vi "Lithography.vi"(8 "Enum":enum16{"Stop", "Start"}(ring), 10 "error in (no error)":errorcluster) -> (2 "error out":errorcluster)   [LabVIEW 2014]
panel:
  in  "AutoItX3Lib.IAutoItX3":refnum<k7>
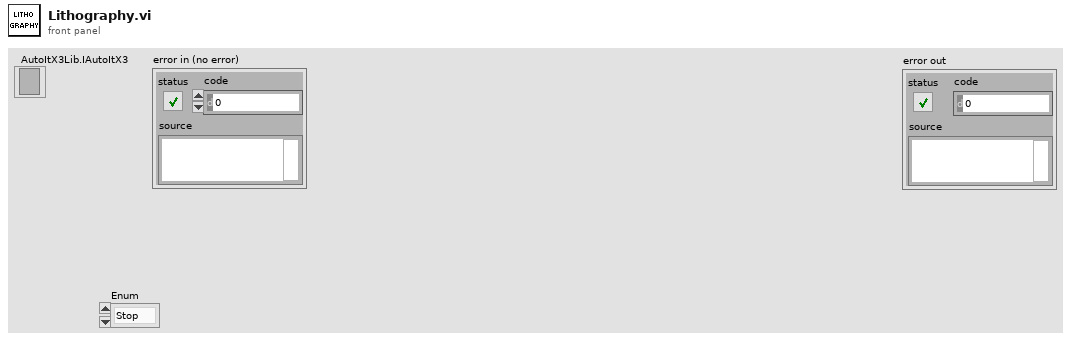
[diagram p1: front panel]
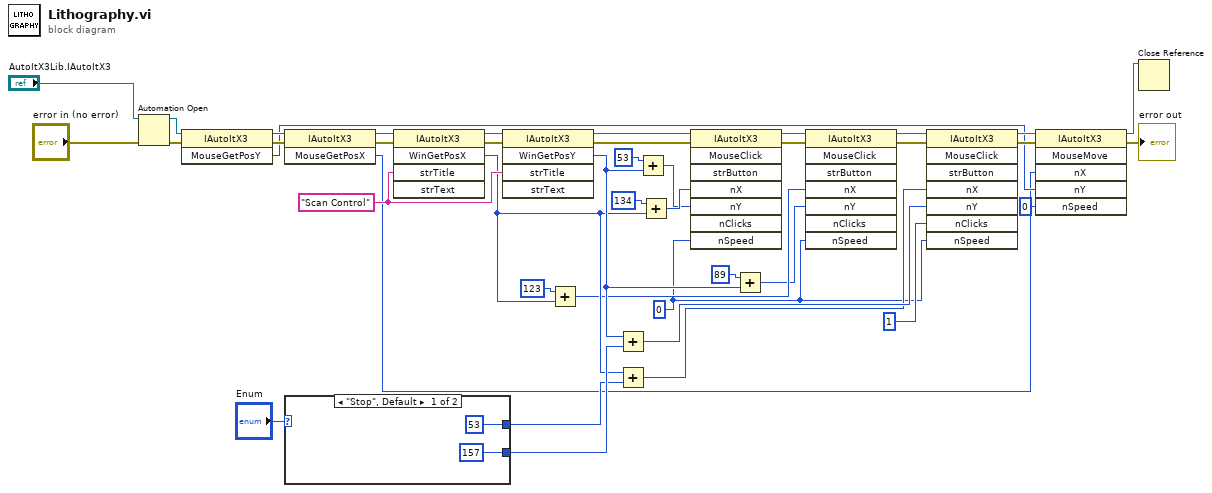
[diagram p0: block diagram]
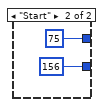
[diagram p2: hidden frame]
diagram:
  w10 = 0 ("nSpeed")
  w37 = "Scan Control" ("strTitle")
  n1 = Automation Open(error in (no error)="error in (no error)", Automation Refnum="AutoItX3Lib.IAutoItX3") -> (Automation Refnum=w39:refnum<k7>, error out=w4:errorcluster)  [unwired: 2 in]
  n2 = invoke class="IAutoItX3" method="MouseGetPosY"(reference=w39, error in=w4) -> (reference out=w8:refnum<k7>, error out=w5:errorcluster, "MouseGetPosY"=w3:i32)  [unwired: 1 in]
  n3 = invoke class="IAutoItX3" method="MouseGetPosX"(reference=w8, error in=w5) -> (reference out=w9:refnum<k7>, error out=w6:errorcluster, "MouseGetPosX"=w2:i32)  [unwired: 1 in]
  n4 = case shown="\"Stop\", Default" "Enum" {
    tunnel: [157 ("y") 156 ("y")] -> w33
    tunnel: [53 ("y") 75 ("y")] -> w29
    frame "Stop", Default {
    }
    frame "Start" {
    }
  }
  n5 = invoke class="IAutoItX3" method="WinGetPosX"(reference=w9, error in=w6, "strTitle"=w37) -> (reference out=w35:refnum<k7>, error out=w36:errorcluster, "WinGetPosX"=w19:i32)  [unwired: 2 in, 2 out]
  n6 = invoke class="IAutoItX3" method="WinGetPosY"(reference=w35, error in=w36, "strTitle"=w37) -> (reference out=w40:refnum<k7>, error out=w23:errorcluster, "WinGetPosY"=w20:i32)  [unwired: 2 in, 2 out]
  n7 = Add(x=123, y=w19) -> (x+y=w16:i32)
  n8 = Add(x=w20, y=w33) -> (x+y=w34:i32)
  n9 = Add(x=w19, y=w29) -> (x+y=w30:i32)
  n10 = Add(x=53, y=w20) -> (x+y=w17:i32)
  n11 = Add(x=134, y=w19) -> (x+y=w18:i32)
  n12 = invoke class="IAutoItX3" method="MouseClick"(reference=w40, error in=w23, "nX"=w18, "nY"=w17, "nSpeed"=w10) -> (reference out=w25:refnum<k7>, error out=w22:errorcluster)  [unwired: 3 in, 6 out]
  n13 = Add(x=89, y=w20) -> (x+y=w15:i32)
  n14 = invoke class="IAutoItX3" method="MouseClick"(reference=w25, error in=w22, "nX"=w16, "nY"=w15, "nSpeed"=w10) -> (reference out=w24:refnum<k7>, error out=w21:errorcluster)  [unwired: 3 in, 6 out]
  n15 = invoke class="IAutoItX3" method="MouseClick"(reference=w24, error in=w21, "nX"=w30, "nY"=w34, "nClicks"=1, "nSpeed"=w10) -> (reference out=w32:refnum<k7>, error out=w31:errorcluster)  [unwired: 2 in, 6 out]
  n16 = invoke class="IAutoItX3" method="MouseMove"(reference=w32, error in=w31, "nX"=w2, "nY"=w3, "nSpeed"=0) -> (reference out=w7:refnum<k7>, error out=→"error out":errorcluster)  [unwired: 1 in, 4 out]
  n17 = Close Reference(reference=w7) -> ()  [unwired: 1 in, 1 out]
